vi "Mnist_Pic2Arr.vi"(11 "empty picture":picture) -> (3 "Img 8 bit":i64[][](array[numeric]))   [LabVIEW 2018]
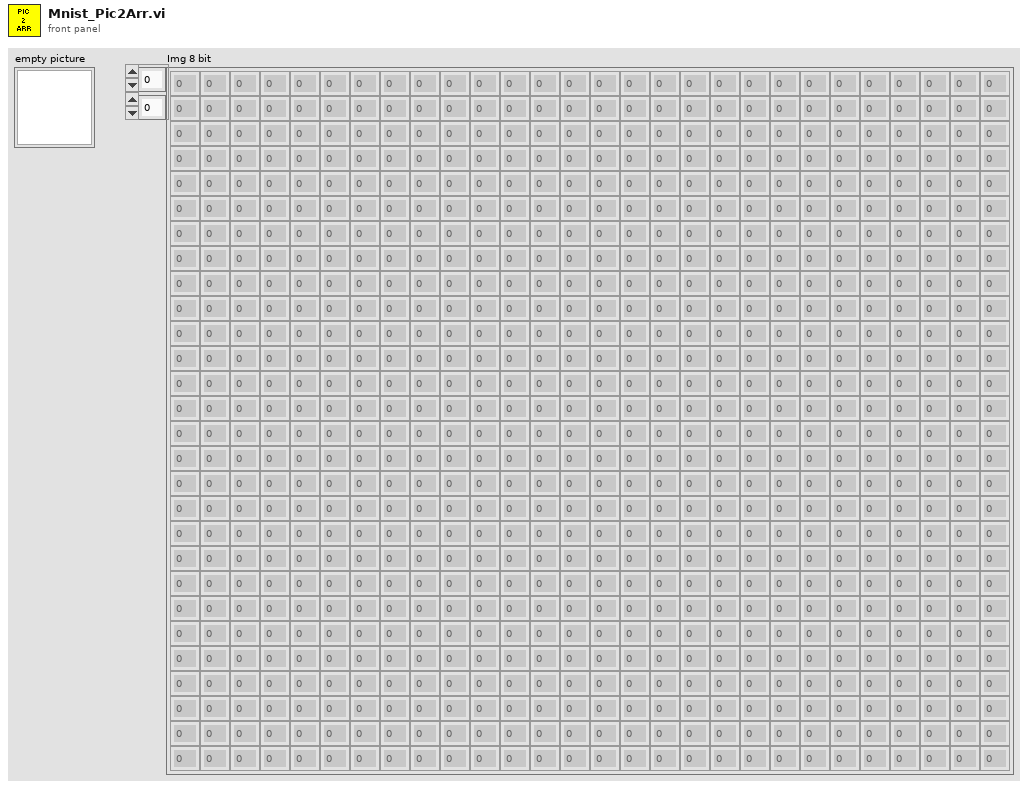
[diagram p1: front panel]
types:
  T1 = typedef "imagedata.ctl" = cluster{"image type":i32, "image depth":i32, "image":u8[], "mask":u8[], "colors":u32[], "Rectangle":cluster{"left":i16, "top":i16, "right":i16, "bottom":i16}}
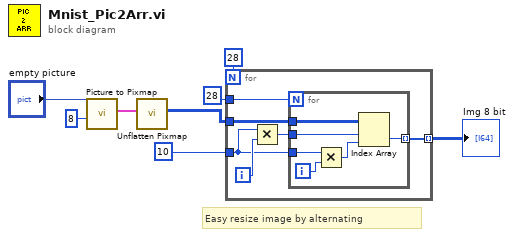
[diagram p0: block diagram]
diagram:
  # "Easy resize image by alternating"
  n1 = call <vilib>:"Picture to Pixmap.vi"("depth"=8, "picture"="empty picture") -> ("image data"=w4:T1)  [unwired: 8 in, 1 out]
  n2 = call <vilib>:"Unflatten Pixmap.vi"("image data"=w4) -> ("8-bit pixmap"=w7:u8[][])  [unwired: 4 in, 6 out]
  n3 = for {
    N: i64 28 -> [_]
    tunnel: w7 -> [w14]
    tunnel: [w13] -> w8 mode=indexing
    tunnel: i64 28 -> [w11]
    tunnel: 10 ("y") -> [w9]
    i -> [w10]
    n4 = Multiply(x=w9, y=w10) -> (x*y=w12:i32)
    n5 = for {
      N: w11 -> [_]
      tunnel: w14 -> [w20]
      tunnel: [w18] -> w13 mode=indexing
      tunnel: w12 -> [w19]
      tunnel: w9 -> [w16]
      i -> [w15]
      n6 = Multiply(x=w16, y=w15) -> (x*y=w17:i32)
      n7 = Index Array(array=w20, index (row)=w19, index (col)=w17) -> (element=w18:u8)
    }
  }
  "Img 8 bit" <- w8
